vi "Open FPGA Ref_No Run.vi"(8 "error in (no error)":errorcluster, 10 "resource name":string, 11 "starter kit host 1.0 in":refnum<class "NI_Robotics_Starter Kit Host_FPGA_1.0.lvclass">) -> (0 "error out":errorcluster, 2 "FPGA Interface":T1, 3 "starter kit host 1.0 out":refnum<class "NI_Robotics_Starter Kit Host_FPGA_1.0.lvclass">)   [LabVIEW 2017, in "NI_Robotics_Starter Kit Host_FPGA_1.0.lvclass"]
uses:
  <vilib>/robotics/Starter Kit/1.0/FPGA Host Interface/NI_Robotics_Starter Kit Host_FPGA_1.0.lvclass
  <vilib>/robotics/Starter Kit/1.0/FPGA Host Interface/FPGA Refnum.ctl
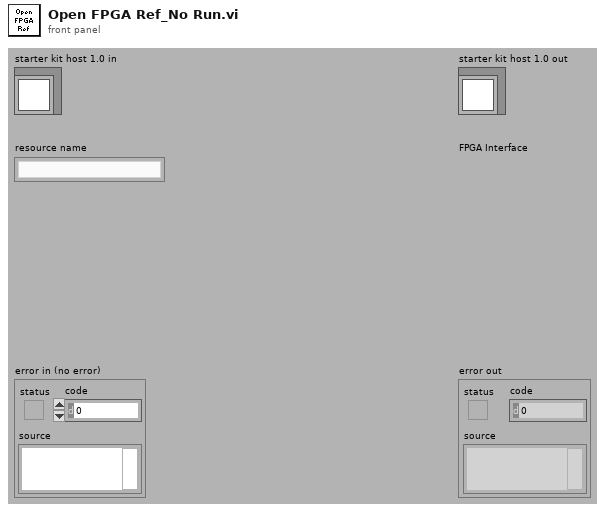
[diagram p1: front panel]
types:
  T1 = typedef "NI_Robotics_Starter Kit Host_FPGA_1.0.lvclass/FPGA Refnum.ctl" = refnum<k20>
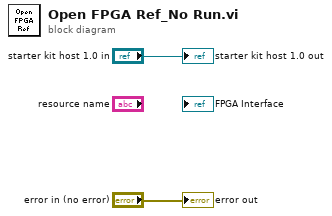
[diagram p0: block diagram]
diagram:
  "error out" <- "error in (no error)"
  "starter kit host 1.0 out" <- "starter kit host 1.0 in"
